vi "Change Motor High Time.vi"(8 "error in":errorcluster, 11 "tCRD in":refnum<class "Open Path CRD.lvclass">) -> (0 "error out":errorcluster, 2 "Filter?":bool, 3 "tCRD out":refnum<class "Open Path CRD.lvclass">)   [LabVIEW 2015, in "Open Path CRD.lvclass"]
doc: "This controls the PWM signal on the servo which is used to open and close the sample line. Most servos operate on a 50 Hz PWM signal, with high times varying between 1-2 ms. Some motors do have endpoints at lower and higher times, but this is a general configuration."
uses:
  Open Path CRD.lvclass
  Open Path CRD.lvclass/Open Path CRD.ctl
  Reusable/Instrument/Instrument.lvclass/Instrument.ctl
  Accessors/Read Servo Switch.vi
  Reusable/Instrument/Read Log Session.vi
  Accessors/Read FPGA Ref.vi
  <vilib>/Utility/error.llb/Error Cluster From Error Code.vi
  <vilib>/rvi/errors/niLvFpgaAdjustHostInterfaceError.vi
  Reusable/CRDS/Main/Read Data.vi
  Reusable/CRDS/Data/Main/Write filter.vi
  Reusable/CRDS/Main/Write Data.vi
  Open Path FPGA Ref.ctl
  <vilib>/rvi/interface/nirviReadWriteControl/nirviReadWriteControl.xnode
  FPGA Bitfiles/Handix_OpenPathCRD.lvbitx
  Reusable/CRDS/Data/Main/CRDS Data.lvclass
  Switch/Servo Switch.lvclass
  <userlib>/_Session Fwk/Session - Root.lvclass
  Reusable/Instrument/Instrument.lvclass
  Reusable/Session Log/System Log.lvclass
  NiFpgaLv.dll
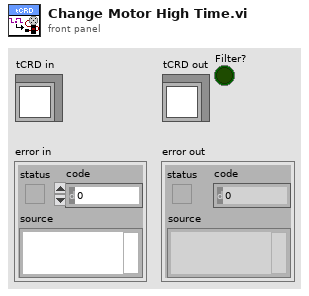
[diagram p1: front panel]
types:
  T1 = typedef "Open Path CRD.lvclass/Open Path FPGA Ref.ctl" = refnum<k20>
  T2 = typedef "Session - Root.lvclass/Session Handle.ctl" = refnum<data-value>
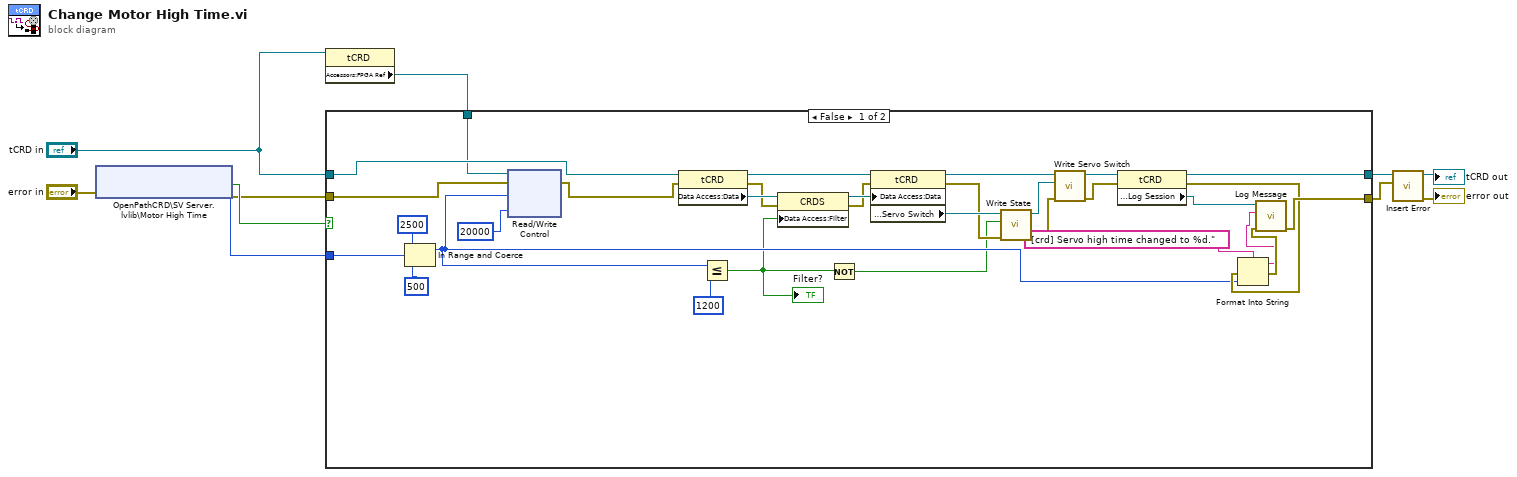
[diagram p0: block diagram]
diagram:
  n1 = shared-variable "OpenPathCRD\\SV Server.lvlib\\Motor High Time"(error in="error in") -> (w9:u32, error out=w8:errorcluster, w10:bool)  [unwired: 1 in]
  n2 = property class="tCRD"(reference="tCRD in") -> ("Accessors:FPGA Ref"=w1:T1)  [unwired: 1 in, 2 out]
  n3 = case shown="False" w10 {
    tunnel: "tCRD in" -> [w40 w43]
    tunnel: [w24 w43] -> w6
    tunnel: w9 -> [w41 _]
    tunnel: w8 -> [w39 w42]
    tunnel: [w23 w42] -> w5
    tunnel: w1 -> [w18 _]
    frame False {
      n4 = In Range and Coerce(upper limit=u32 2500, x=w41, lower limit=u32 500) -> (coerced(x)=w14:u32)  [unwired: 1 out]
      n5 = xnode "Read/Write Control"("FPGA VI Reference In"=w18, "error in"=w39, "High"=w14, "Low"=u32 20000 ("x")) -> ("error out"=w38:errorcluster)  [unwired: 1 out]
      n6 = property class="tCRD"(reference=w40, error in=w38) -> (reference out=w37:refnum<class "Open Path CRD.lvclass">, error out=w33:errorcluster, "Data Access:Data"=w36:refnum<class "CRDS Data.lvclass">)
      n7 = Less Or Equal?(x=w14, y=u32 1200) -> (x <= y?=w13:bool)
      "Filter?" <- w13
      n8 = property class="CRDS"(reference=w36, error in=w33, "Data Access:Filter"=w13) -> (reference out=w35:refnum<class "CRDS Data.lvclass">, error out=w34:errorcluster)
      n9 = Not(x=w13) -> (.not. x?=w11:bool)
      n10 = property class="tCRD"(reference=w37, error in=w34, "Data Access:Data"=w35) -> (reference out=w29:refnum<class "Open Path CRD.lvclass">, error out=w30:errorcluster, "Accessors:Servo Switch"=w31:refnum<class "Servo Switch.lvclass">)
      n11 = call-dynamic "Write State.vi"("error in"=w30, "State"=w11, "Switch in"=w31) -> ("error out"=w28:errorcluster, "Switch out"=w27:refnum<class "Servo Switch.lvclass">)  [unwired: 7 in]
      n12 = call "Write Servo Switch.vi"("error in"=w28, "Servo Switch"=w27, "tCRD in"=w29) -> ("error out"=w25:errorcluster, "tCRD out"=w26:refnum<class "Open Path CRD.lvclass">)  [unwired: 7 in]
      n13 = property class="tCRD"(reference=w26, error in=w25) -> (reference out=w24:refnum<class "Open Path CRD.lvclass">, error out=w21:errorcluster, "Accessors:Log Session"=w12:T2)
      n14 = Format Into String(format string="[crd] Servo high time changed to %d." ("MSG In"), error in=w21, w14) -> (resulting string=w19:string, error out=w20:errorcluster)  [unwired: 1 in]
      n15 = call "Log Message.vi"("error in"=w20, "MSG In"=w19, "session in"=w12) -> ("error out"=w23:errorcluster)  [unwired: 7 in, 1 out]
    }
    frame True {
    }
  }
  n16 = call "Insert Error.vi"("err"=w5, "Instrument in"=w6) -> ("error out"=→"error out":errorcluster, "Instrument out"=→"tCRD out":refnum<class "Open Path CRD.lvclass">)  [unwired: 7 in, 1 out]
